vi "GetQueue.vi"(8 "error in (no error)":errorcluster) -> (0 "error out":errorcluster, 3 "queue out":refnum<queue>)   [LabVIEW 2019, in "AnimatorXControl.xctl"]
uses:
  AnimatorXControl.xctl
  QueueElement.ctl
  AnimatorSettings.ctl
  AnimatorCommand.ctl
panel:
  in  "QueueElement":T1
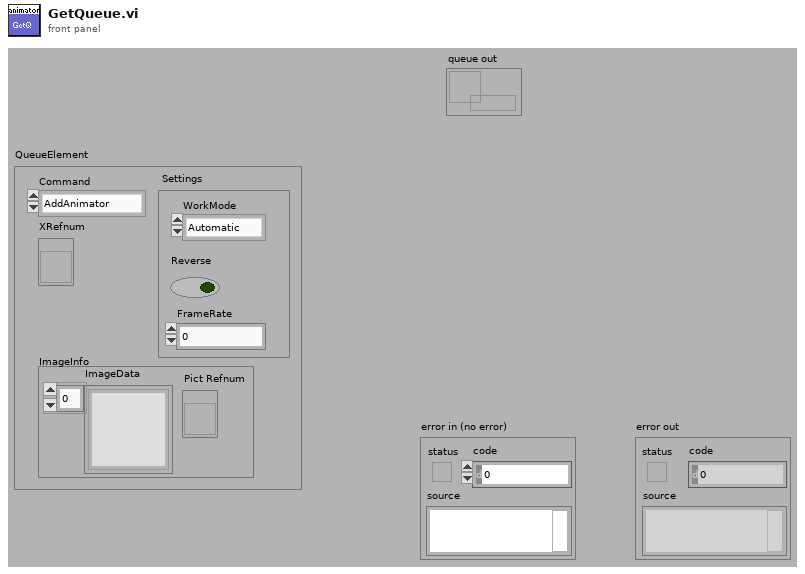
[diagram p1: front panel]
types:
  T1 = typedef "AnimatorXControl.xctl/QueueElement.ctl" = cluster{"Settings":T2, "Command":T3, "ImageInfo":cluster{"ImageData":picture[], "Pict Refnum":refnum<vi>}, "XRefnum":refnum<vi>}
  T2 = typedef "AnimatorXControl.xctl/AnimatorSettings.ctl" = cluster{"Reverse":bool, "FrameRate":dbl, "WorkMode":enum16{"Automatic", "UseValue"}}
  T3 = typedef "AnimatorXControl.xctl/AnimatorCommand.ctl" = enum16{"AddAnimator", "RemoveAnimator", "Settings"}
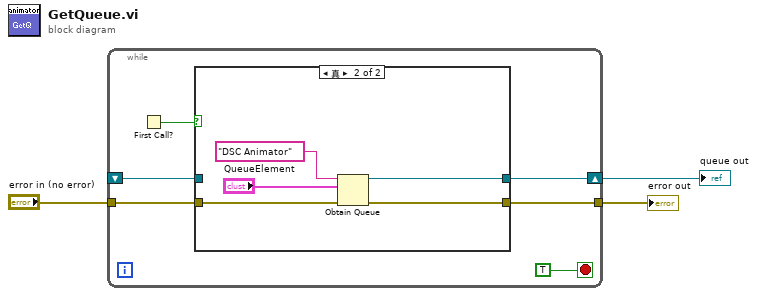
[diagram p0: block diagram]
diagram:
  n1 = while {
    tunnel: "error in (no error)" -> [w8]
    tunnel: [w7] -> w2
    shift-right: [w6] -> w1
    shift-left: _ -> [w5]
    stop <- TRUE stop-if-true
    n2 = First Call?() -> (First Call?: T/F=w4:bool)
    n3 = case shown="真" w4 {
      tunnel: w8 -> [w11 w14]
      tunnel: [w11 w13] -> w7
      tunnel: [w10 w12] -> w6
      tunnel: w5 -> [w10 _]
      frame False {
      }
      frame True {
        n4 = Obtain Queue(name (unnamed)="DSC Animator", element data type="QueueElement", error in (no error)=w14) -> (queue out=w12:refnum<queue>, error out=w13:errorcluster)  [unwired: 2 in, 1 out]
      }
    }
  }
  "error out" <- w2
  "queue out" <- w1
